vi "NI-XNET Monitor Init.vi"(8 "Error In":errorcluster, 10 "Parameters":variant, 11 "Data Access Engine in":refnum<class "Data Access Engine.lvclass">) -> (0 "Error Out":errorcluster, 3 "Process  Data Out":T1, 4 "Async Loop Rate (s)":dbl)   [LabVIEW 2017, in "NI-XNET Monitor Engine.lvlib"]
uses:
  NI-XNET Monitor Engine.lvlib
  <vilib>/NI/NIVS Inline Async API/_Data Access Engine/Data Access Engine/Data Access Engine.lvclass
  RTMonitorRefnums.ctl
  <vilib>/NI/NIVS Inline Async API/_Data Access Engine/Data Access Engine/Types/Write.DVR.ctl
  <vilib>/NI/NIVS Inline Async API/_Data Access Engine/Access Type Classes/Write/Write.lvclass
  Shared/Compiled.Data.ctl
  <vilib>/NI/NIVS Inline Async API/_Data Access Engine/Data Access Engine/Methods/Write.Lookup.vi
  Shared/NI-XNET Monitor Shared.lvlib
  <vilib>/NI VeriStand/Custom Device Tools/Custom Device Utility Library/Custom Device Utility Library.lvlib
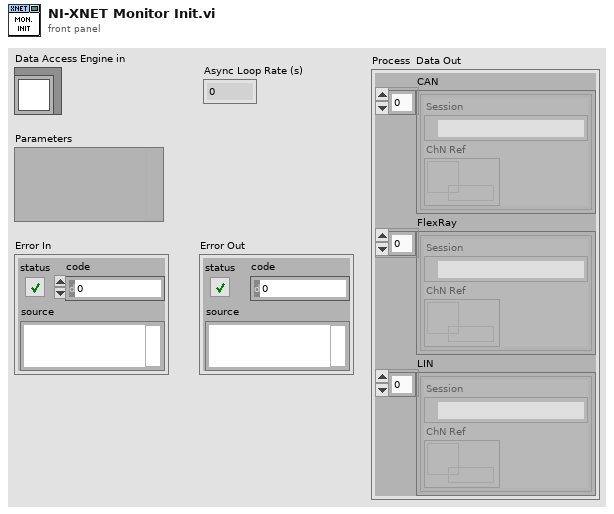
[diagram p1: front panel]
types:
  T1 = typedef "NI-XNET Monitor Engine.lvlib/RTMonitorRefnums.ctl" = cluster{"CAN":cluster{"Session":refnum<k21>, "ChN Ref":T2}[], "FlexRay":cluster{"Session":refnum<k21>, "ChN Ref":T2}[], "LIN":cluster{"Session":refnum<k21>, "ChN Ref":T2}[]}
  T2 = typedef "Data Access Engine.lvlib/Data Access Engine.lvclass/Write.DVR.ctl" = refnum<data-value>
  T3 = typedef "NI-XNET Monitor Shared.lvlib/Compiled.Data.ctl" = cluster{"CAN":string[], "FlexRay":string[], "LIN":string[], "Async Loop Rate (s)":dbl}
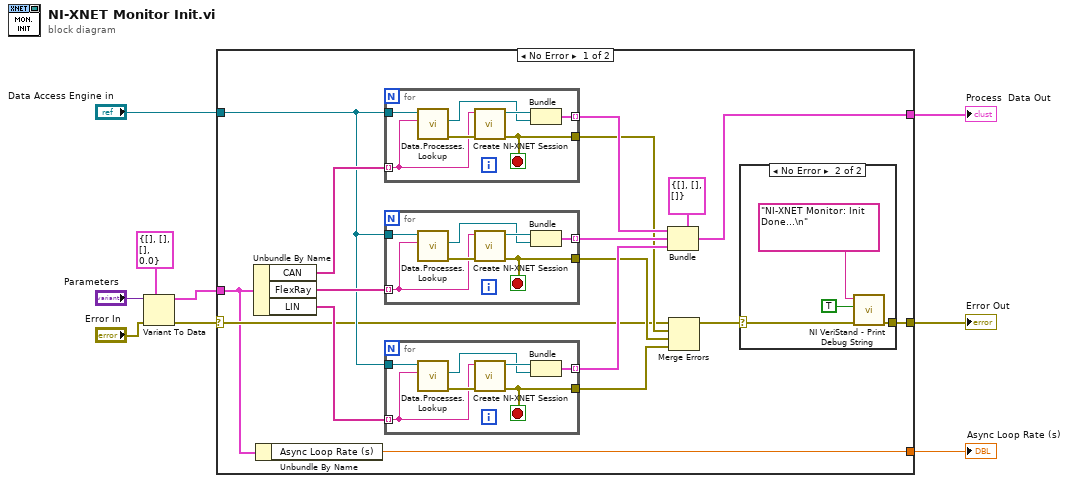
[diagram p0: block diagram]
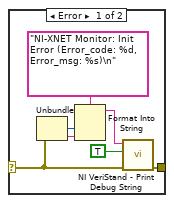
[diagram p2: hidden frame]
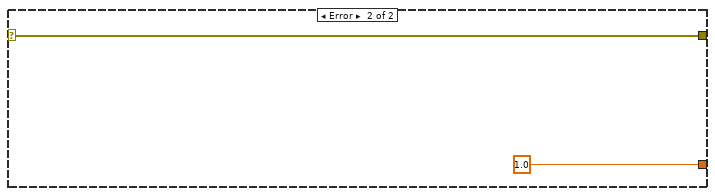
[diagram p3: hidden frame]
diagram:
  n1 = Variant To Data(error in="Error In", type=T3 {"CAN"=[], "FlexRay"=[], "LIN"=[], "Async Loop Rate (s)"=0.0} ("Compiled.Data"), Variant="Parameters") -> (data=w3:T3, error out=w4:errorcluster)
  n2 = case shown="No Error" w4 {
    selector: w4 -> [w15 w60]
    tunnel: w3 -> [w13 _]
    tunnel: "Data Access Engine in" -> [w23 _]
    tunnel: [w19 _] -> w9
    tunnel: [w10 w60] -> w5
    tunnel: [w12 1.0 ("Async Loop Rate (s)")] -> w1
    frame No Error {
      n3 = Unbundle By Name(w13) -> ("CAN"=w26:string[], "FlexRay"=w24:string[], "LIN"=w25:string[])
      n4 = Unbundle By Name(w13) -> ("Async Loop Rate (s)"=w12:dbl)
      n5 = for {
        tunnel: w26 -> [w56] mode=indexing
        tunnel: w23 -> [w58]
        tunnel: [w55] -> w16
        tunnel: [w52] -> w22 mode=indexing
        stop <- w55 stop-if-true
        n6 = call-poly <vilib>:"Data.Processes.Lookup.vi"("Name"=w56, "Data Access API in"=w58) -> ("error out"=w57:errorcluster, "Ref"=w53:T2)  [unwired: 6 in, 2 out]
        n7 = call "Create NI-XNET Session.vi"("Error In"=w57, "NI-XNET Port In"=w56) -> ("Error Out"=w55:errorcluster, "Session out"=w54:refnum<k21>)  [unwired: 8 in]
        n8 = Bundle("Session out"=w54, "Ref"=w53) -> (w52:cluster{"Session out":refnum<k21>, "Ref":T2})  [unwired: 1 in]
      }
      n9 = for {
        tunnel: w24 -> [w49] mode=indexing
        tunnel: w23 -> [w51]
        tunnel: [w48] -> w17
        tunnel: [w45] -> w21 mode=indexing
        stop <- w48 stop-if-true
        n10 = call-poly <vilib>:"Data.Processes.Lookup.vi"("Name"=w49, "Data Access API in"=w51) -> ("error out"=w50:errorcluster, "Ref"=w46:T2)  [unwired: 6 in, 2 out]
        n11 = call "Create NI-XNET Session.vi"("Error In"=w50, "NI-XNET Port In"=w49) -> ("Error Out"=w48:errorcluster, "Session out"=w47:refnum<k21>)  [unwired: 8 in]
        n12 = Bundle("Session out"=w47, "Ref"=w46) -> (w45:cluster{"Session out":refnum<k21>, "Ref":T2})  [unwired: 1 in]
      }
      n13 = for {
        tunnel: w25 -> [w42] mode=indexing
        tunnel: w23 -> [w44]
        tunnel: [w41] -> w18
        tunnel: [w38] -> w20 mode=indexing
        stop <- w41 stop-if-true
        n14 = call-poly <vilib>:"Data.Processes.Lookup.vi"("Name"=w42, "Data Access API in"=w44) -> ("error out"=w43:errorcluster, "Ref"=w39:T2)  [unwired: 6 in, 2 out]
        n15 = call "Create NI-XNET Session.vi"("Error In"=w43, "NI-XNET Port In"=w42) -> ("Error Out"=w41:errorcluster, "Session out"=w40:refnum<k21>)  [unwired: 8 in]
        n16 = Bundle("Session out"=w40, "Ref"=w39) -> (w38:cluster{"Session out":refnum<k21>, "Ref":T2})  [unwired: 1 in]
      }
      n17 = Bundle(cluster=T1 {"CAN"=[], "FlexRay"=[], "LIN"=[]}, "CAN"=w22, "FlexRay"=w21, "LIN"=w20) -> (w19:T1)
      n18 = Merge Errors(w15, w16, w17, w18) -> (w11:errorcluster)
      n19 = case shown="No Error" w11 {
        selector: w11 -> [w28 w36]
        tunnel: [w27 w35] -> w10
        frame Error {
          n20 = Unbundle(w28) -> ("code"=w32:i32, "source"=w33:string)  [unwired: 1 out]
          n21 = Format Into String(format string="NI-XNET Monitor: Init Error (Error_code: %d, Error_msg: %s)\n" ("Message"), w32, w33) -> (resulting string=w31:string)  [unwired: 2 in, 1 out]
          n22 = call <vilib>:"NI VeriStand - Print Debug String.vi"("error in (no error)"=w28, "Add to log file? (T)"=TRUE, "Message"=w31) -> ("error out"=w27:errorcluster)  [unwired: 8 in]
        }
        frame No Error {
          n23 = call <vilib>:"NI VeriStand - Print Debug String.vi"("error in (no error)"=w36, "Add to log file? (T)"=TRUE, "Message"="NI-XNET Monitor: Init Done...\n") -> ("error out"=w35:errorcluster)  [unwired: 8 in]
        }
      }
    }
    frame Error {
    }
  }
  "Error Out" <- w5
  "Process  Data Out" <- w9
  "Async Loop Rate (s)" <- w1
